vi "JLink Utility.vi"(6 "run minimized? (F)":bool, 7 "wait until completion? (T)":bool=TRUE, 8 "error in (no error)":errorcluster, 10 "Parameters String":string, 11 "JLink Directory":path) -> (0 "error out":errorcluster, 2 "standard output":string)   [LabVIEW 2016, in "JLink Commander.lvlib"]
doc: "This VI serves as a JFlash Command Prompt / CLI by accepting and passing command to JFlash.exe."
uses:
  JLink Commander.lvlib
panel:
  out "return code":i32
  out "length":i32
  out "command line":string
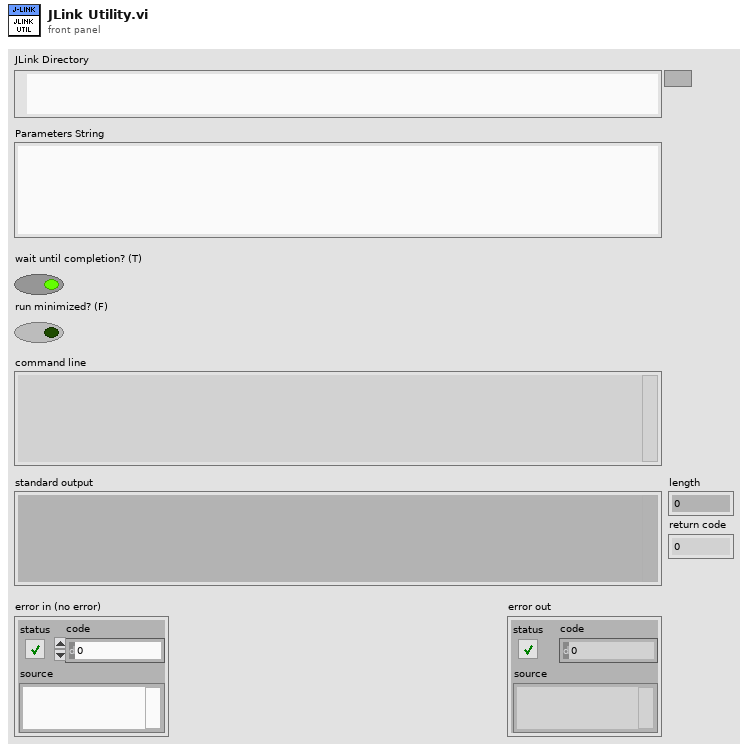
[diagram p1: front panel]
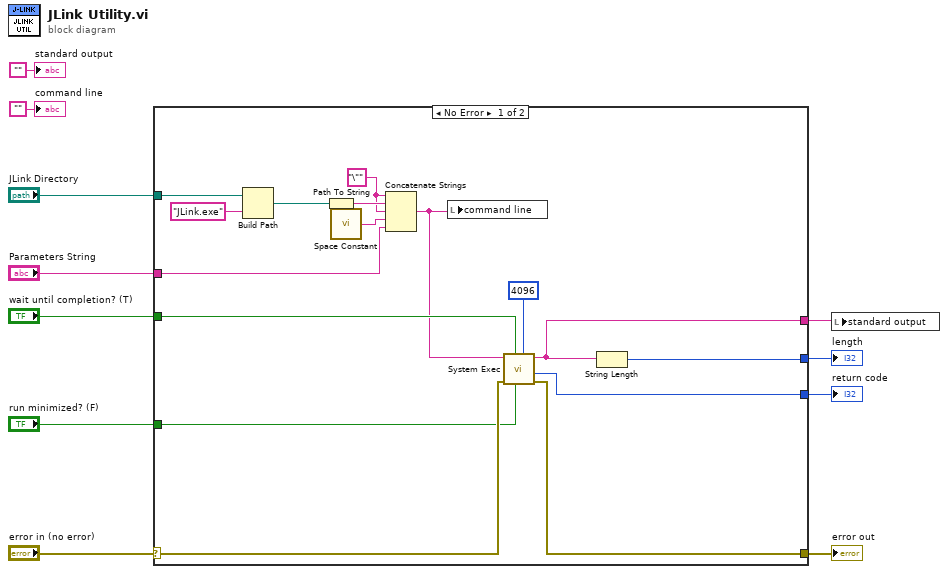
[diagram p0: block diagram]
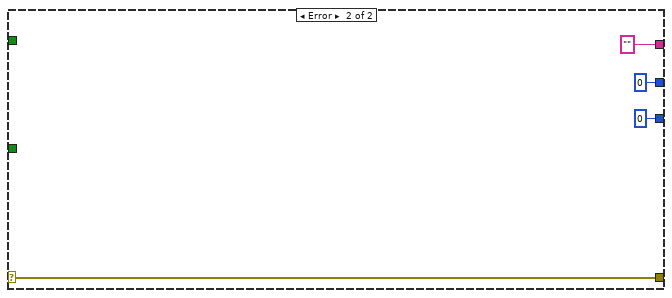
[diagram p2: hidden frame]
diagram:
  n1 = case shown="No Error" "error in (no error)" {
    selector: "error in (no error)" -> [w26 w31]
    tunnel: [w25 w31] -> w10
    tunnel: "JLink Directory" -> [w17 _]
    tunnel: [w21 "" ("standard output")] -> w4
    tunnel: "wait until completion? (T)" -> [w23 _]
    tunnel: "run minimized? (F)" -> [w22 _]
    tunnel: "Parameters String" -> [w13 _]
    tunnel: [w20 0] -> w3
    tunnel: [w19 0 ("return code")] -> w2
    frame No Error {
      w14 = "\"" ("string")
      n2 = Build Path(base path=w17, name or relative path="JLink.exe" ("string")) -> (appended path=w15:path)
      n3 = Path To String(path=w15) -> (string=w27:string)
      n4 = call <vilib>:"Space Constant.vi"() -> ("String"=w12:string)
      n5 = Concatenate Strings(w14, w27, w14, w12, w13) -> (w18:string)
      n6 = local write "command line"(w18) -> ()
      n7 = call <vilib>:"System Exec.vi"("expected output size  (4096)"=u32 4096, "run minimized? (F)"=w22, "wait until completion? (T)"=w23, "error in (no error)"=w26, "command line"=w18) -> ("error out"=w25:errorcluster, "return code"=w19:i32, "standard output"=w21:string)  [unwired: 3 in, 1 out]
      n8 = String Length(string=w21) -> (length=w20:i32)
    }
    frame Error {
    }
  }
  "error out" <- w10
  "length" <- w3
  "return code" <- w2
  n9 = local write "standard output"(w4) -> ()
  "standard output" <- ""
  "command line" <- ""
